vi "AIT 664 - Create Default Message Buffers.vi"(0 "Parameter Driver Data in":T1 {"Num Bits" min=1 max=32}) -> (4 "Default Message Data out":u8[](array[numeric]))   [LabVIEW 2013, in "AIT 664 Custom Device.lvlib"]
doc: "Create default message data for given channels"
uses:
  AIT 664 Custom Device.lvlib
  RT Controls/AIT 664 - Driver Data.ctl
  Controls and Global/Start Bit.ctl
  Controls and Global/Number of Bits.ctl
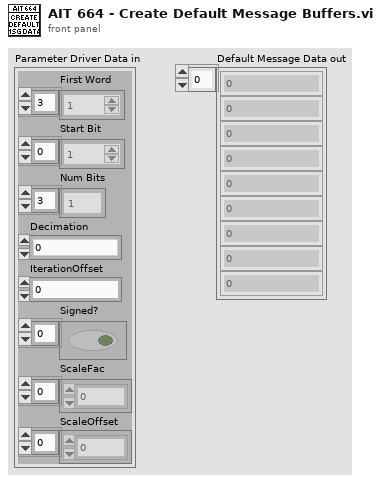
[diagram p1: front panel]
types:
  T1 = typedef "AIT 664 Custom Device.lvlib/AIT 664 - Driver Data.ctl" = cluster{"First Word":T2[], "Start Bit":T2[], "Num Bits":T3[], "Decimation":i32, "IterationOffset":i32, "Signed?":bool[], "ScaleFac":dbl[], "ScaleOffset":dbl[]}
  T2 = typedef "AIT 664 Custom Device.lvlib/Start Bit.ctl" = i32
  T3 = typedef "AIT 664 Custom Device.lvlib/Number of Bits.ctl" = i32
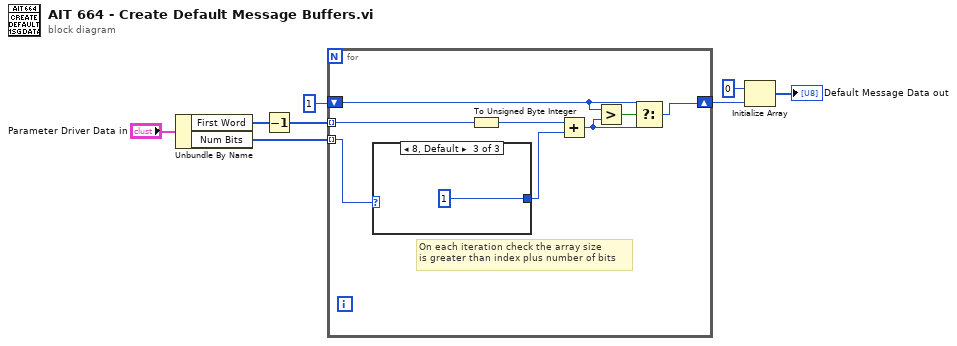
[diagram p0: block diagram]
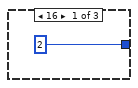
[diagram p2: hidden frame]
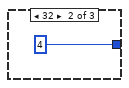
[diagram p3: hidden frame]
diagram:
  n1 = Unbundle By Name("Parameter Driver Data in") -> ("First Word"=w6:T2[], "Num Bits"=w7:T3[])
  n2 = Decrement(x=w6) -> (x-1=w5:T2[])
  n3 = for {
    shift-right: [w9] -> w3
    shift-left: u8 1 ("dimension size") -> [w11]
    tunnel: w5 -> [w14] mode=indexing
    tunnel: w7 -> [w16] mode=indexing
    # "On each iteration check the array size\nis greater than index plus number of bits"
    n4 = case shown="8, Default" w16 {
      tunnel: [u8 2 ("dimension size") u8 4 ("dimension size") u8 1 ("dimension size")] -> w15
      frame 16 {
      }
      frame 32 {
      }
      frame 8, Default {
      }
    }
    n5 = To Unsigned Byte Integer(number=w14) -> (unsigned 8bit integer=w13:u8)
    n6 = Add(x=w13, y=w15) -> (x+y=w10:u8)
    n7 = Greater?(x=w11, y=w10) -> (0:w12:bool)
    n8 = Select(t=w11, s=w12, f=w10) -> (s? t:f=w9:u8)
  }
  n9 = Initialize Array(u8 0 ("dimension size"), w3) -> (→"Default Message Data out":u8[])
